vi "NewFlexUIActorLibrary.vi"(8 "error in (no error)":errorcluster, 11 "FlexUIActorMaker in":refnum<class "FlexUIActorMaker.lvclass">) -> (0 "error out":errorcluster, 3 "FlexUIActorMaker out":refnum<class "FlexUIActorMaker.lvclass">)   [LabVIEW 2016, in "FlexUIActorMaker.lvlib" / "FlexUIActorMaker.lvclass"]
uses:
  FlexUIActorMaker.lvclass
  FlexUIActorMaker.lvclass/FlexUIActorMaker.ctl
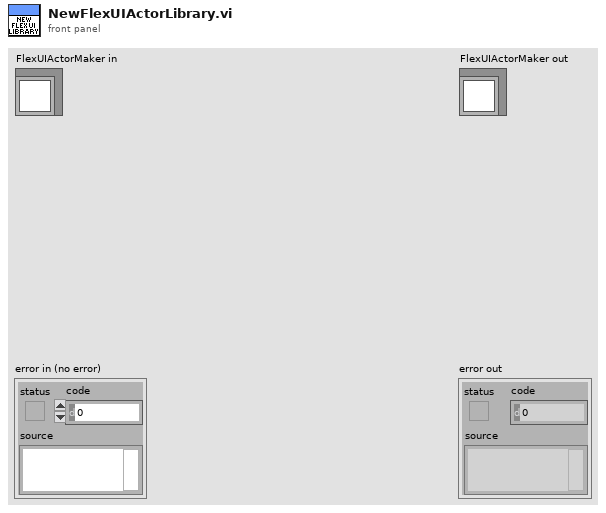
[diagram p1: front panel]
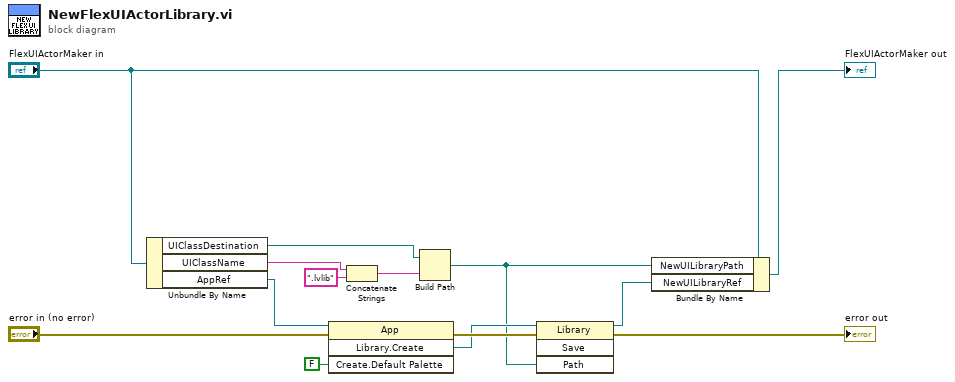
[diagram p0: block diagram]
diagram:
  n1 = Unbundle By Name("FlexUIActorMaker in") -> ("UIClassDestination"=w5:path, "UIClassName"=w4:string, "AppRef"=w8:refnum<vi>)
  n2 = invoke class="App" method="Library.Create"(reference=w8, error in="error in (no error)", "Create.Default Palette"=FALSE ("Create:Default Palette")) -> (error out=w13:errorcluster, "Create Library"=w9:refnum<vi>)  [unwired: 1 in, 2 out]
  n3 = Concatenate Strings(w4, ".lvlib" ("string")) -> (w2:string)
  n4 = Build Path(base path=w5, name or relative path=w2) -> (appended path=w1:path)
  n5 = invoke class="Library" method="Save"(reference=w9, error in=w13, "Path"=w1) -> (reference out=w7:refnum<vi>, error out=→"error out":errorcluster)  [unwired: 1 in, 2 out]
  n6 = Bundle By Name(cluster="FlexUIActorMaker in", "NewUILibraryPath"=w1, "NewUILibraryRef"=w7) -> (→"FlexUIActorMaker out":refnum<class "FlexUIActorMaker.lvclass">)
